vi "Configure ARB Sequence Pacing.vi"(8 "error in":errorcluster, 10 "Type":u16(ring) items=["DWELl", "TRIG"], 11 "VISA resource name":refnum<visa-resource-name>) -> (0 "error out":errorcluster, 3 "VISA resource name out":refnum<visa-resource-name>)   [LabVIEW 2015, in "IT-M3900C.lvlib"]
doc: "The command to set the sequence contains multiple waveform, the waveform when switching, and pacing control bits and TOUT set to TRIG waveform switch sends a trigger signal is needed to continue to run a waveform, set to DWELl time by IO4 mouth (configured to TOUT) to produce pulse signal.\n<b>Type</b>\n0: DWELl\n1: TRIG"
uses:
  <instrlib>/IT-M3900C/IT-M3900C.lvlib
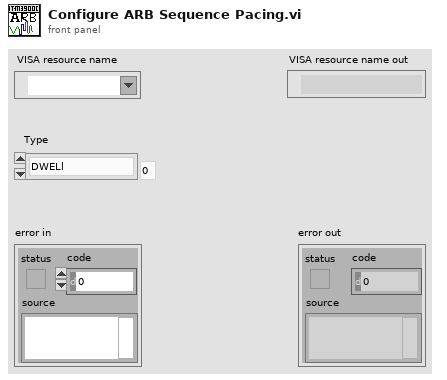
[diagram p1: front panel]
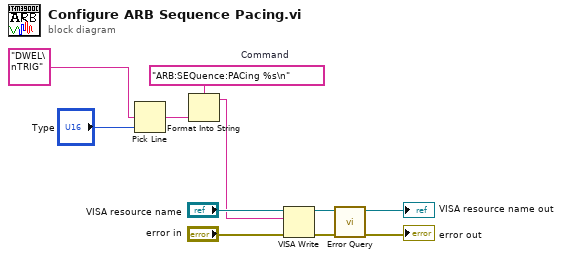
[diagram p0: block diagram]
diagram:
  w5 = "ARB:SEQuence:PACing %s\n"  # Command
  n1 = Pick Line(multi-line string="DWEL\nTRIG", line index="Type") -> (output string=w1:string)  [unwired: 1 in]
  n2 = Format Into String(format string=w5, w1) -> (resulting string=w4:string)  [unwired: 2 in, 1 out]
  n3 = VISA Write(VISA resource name="VISA resource name", write buffer=w4, error in (no error)="error in") -> (VISA resource name out=w8:refnum<visa-resource-name>, error out=w9:errorcluster)  [unwired: 1 out]
  n4 = call <instrlib>:"Error Query.vi"("error in"=w9, "VISA resource name"=w8) -> ("error out"=→"error out":errorcluster, "VISA resource name out"=→"VISA resource name out":refnum<visa-resource-name>)  [unwired: 6 in, 2 out]
